vi "Build Variable Header Publish.vi"(8 "error in (no error)":errorcluster, 9 "Message ID":u16=1 format="%x", 10 "Topic Name":string="Topic", 11 "QoS":T1(ring)) -> (0 "error out":errorcluster, 2 "Variable Header":u8[](array[numeric]) format="%x")   [LabVIEW 2020, in "DAQIO MQTT.lvlib"]
uses:
  DAQIO MQTT.lvlib
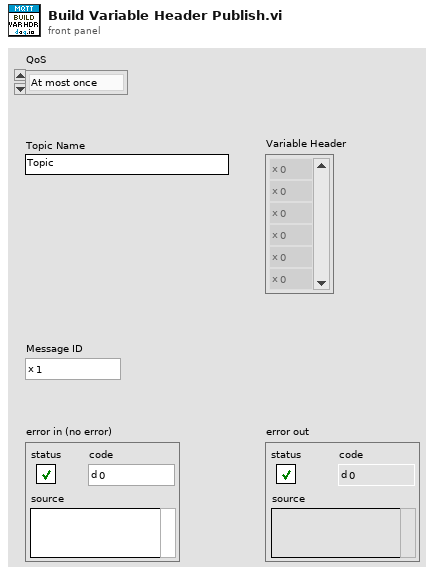
[diagram p1: front panel]
types:
  T1 = enum8{"At most once", "At least once", "Exactly once", "Reserved"}
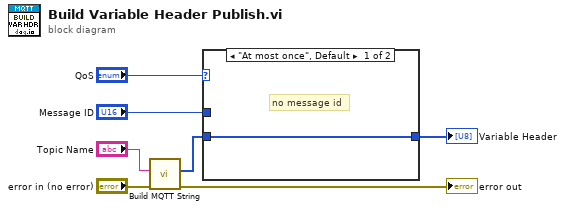
[diagram p0: block diagram]
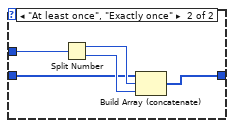
[diagram p2: hidden frame]
diagram:
  n1 = call "Build MQTT String.vi"("error in (no error)"="error in (no error)", "String to be encoded"="Topic Name") -> ("error out"=→"error out":errorcluster, "UTF8 Byte Array"=w3:u8[])  [unwired: 8 in]
  n2 = case shown="\"At most once\", Default" "QoS" {
    tunnel: w3 -> [w8 w9]
    tunnel: [w8 w12] -> w2
    tunnel: "Message ID" -> [_ w13]
    frame "At most once", Default {
      # "no message id"
    }
    frame "At least once", "Exactly once" {
      n3 = Split Number(x=w13) -> (hi(x)=w11:u8, lo(x)=w10:u8)
      n4 = Build Array (concatenate)(w9, w11, w10) -> (w12:u8[])
    }
  }
  "Variable Header" <- w2
